vi "Base32 to Base10.vi"(1 "Base 32":string) -> (0 "Decimal":u64)   [LabVIEW 2016]
uses:
  Printing/Printing.lvlib
panel:
  out "length":i32
  out "Array":u64[](array[numeric])
  out "Array of Strings":string[](array[string])
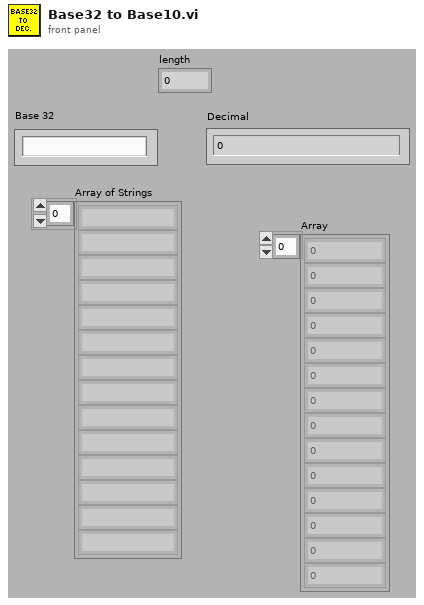
[diagram p1: front panel]
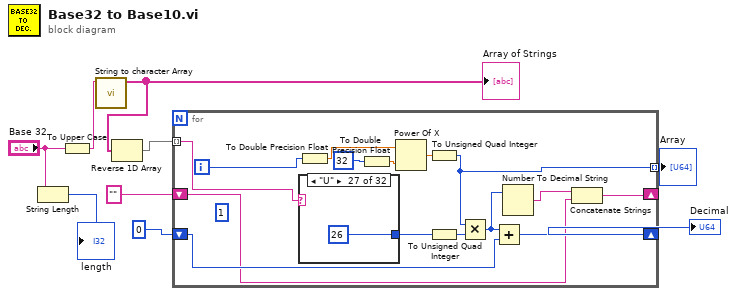
[diagram p0: block diagram]
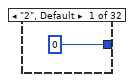
[diagram p2: hidden frame]
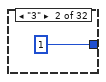
[diagram p3: hidden frame]
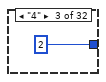
[diagram p4: hidden frame]
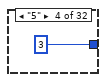
[diagram p5: hidden frame]
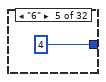
[diagram p6: hidden frame]
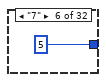
[diagram p7: hidden frame]
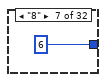
[diagram p8: hidden frame]
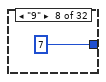
[diagram p9: hidden frame]
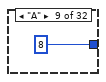
[diagram p10: hidden frame]
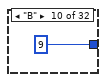
[diagram p11: hidden frame]
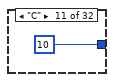
[diagram p12: hidden frame]
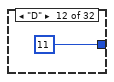
[diagram p13: hidden frame]
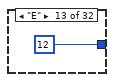
[diagram p14: hidden frame]
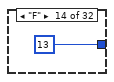
[diagram p15: hidden frame]
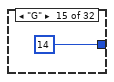
[diagram p16: hidden frame]
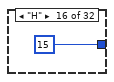
[diagram p17: hidden frame]
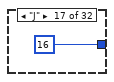
[diagram p18: hidden frame]
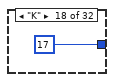
[diagram p19: hidden frame]
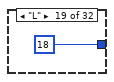
[diagram p20: hidden frame]
diagram:
  n1 = String Length(string="Base 32") -> (length=→"length":i32)
  n2 = To Upper Case(1:"Base 32") -> (0:w7:string)
  n3 = call "String to character Array.vi"("String"=w7) -> ("Array"=w6:string[])  [unwired: 10 in]
  "Array of Strings" <- w6
  n4 = Reverse 1D Array(array=w6) -> (reversed array=w5:string[])
  n5 = for {
    shift-right: [w20] -> w8
    shift-left: u64 0 -> [w21]
    tunnel: w5 -> [w14] mode=indexing
    tunnel: [w15] -> w4 mode=indexing
    shift-right: [w10] -> _
    shift-left: "" -> [w11]
    i -> [w16]
    (unwired) 1 ("length (rest)")
    n6 = case shown="\"U\"" w14 {
      tunnel: [0 1 2 3 4 5 6 7 8 9 10 11 12 13 14 15 16 17 18 19 20 21 22 23 24 25 26 27 28 29 30 31] -> w24
      frame "2", Default {
      }
      frame "3" {
      }
      frame "4" {
      }
      frame "5" {
      }
      frame "6" {
      }
      frame "7" {
      }
      frame "8" {
      }
      frame "9" {
      }
      frame "A" {
      }
      frame "B" {
      }
      frame "C" {
      }
      frame "D" {
      }
      frame "E" {
      }
      frame "F" {
      }
      frame "G" {
      }
      frame "H" {
      }
      frame "J" {
      }
      frame "K" {
      }
      frame "L" {
      }
      frame "M" {
      }
      frame "N" {
      }
      frame "P" {
      }
      frame "Q" {
      }
      frame "R" {
      }
      frame "S" {
      }
      frame "T" {
      }
      frame "U" {
      }
      frame "V" {
      }
      frame "W" {
      }
      frame "X" {
      }
      frame "Y" {
      }
      frame "Z" {
      }
    }
    n7 = To Double Precision Float(number=w16) -> (double precision float=w17:dbl)
    n8 = To Double Precision Float(number=32 ("x")) -> (double precision float=w19:dbl)
    n9 = Power Of X(1:w19, 2:w17) -> (0:w23:dbl)
    n10 = To Unsigned Quad Integer(1:w23) -> (0:w15:u64)
    n11 = To Unsigned Quad Integer(1:w24) -> (0:w22:u64)
    n12 = Multiply(x=w15, y=w22) -> (x*y=w13:u64)
    n13 = Add(x=w13, y=w21) -> (x+y=w20:u64)
    n14 = Number To Decimal String(number=w13) -> (decimal integer string=w12:string)  [unwired: 1 in]
    n15 = Concatenate Strings(w12, w11) -> (w10:string)
  }
  "Decimal" <- w8
  "Array" <- w4
